vi "Ping.vi"(2 "error in":errorcluster caption="错误输入（无错误）", 3 "NetAdress":string) -> (0 "error out":errorcluster caption="错误输出", 1 "Acess":bool)   [LabVIEW 2013]
panel:
  out "standard output":string caption="标准输出"
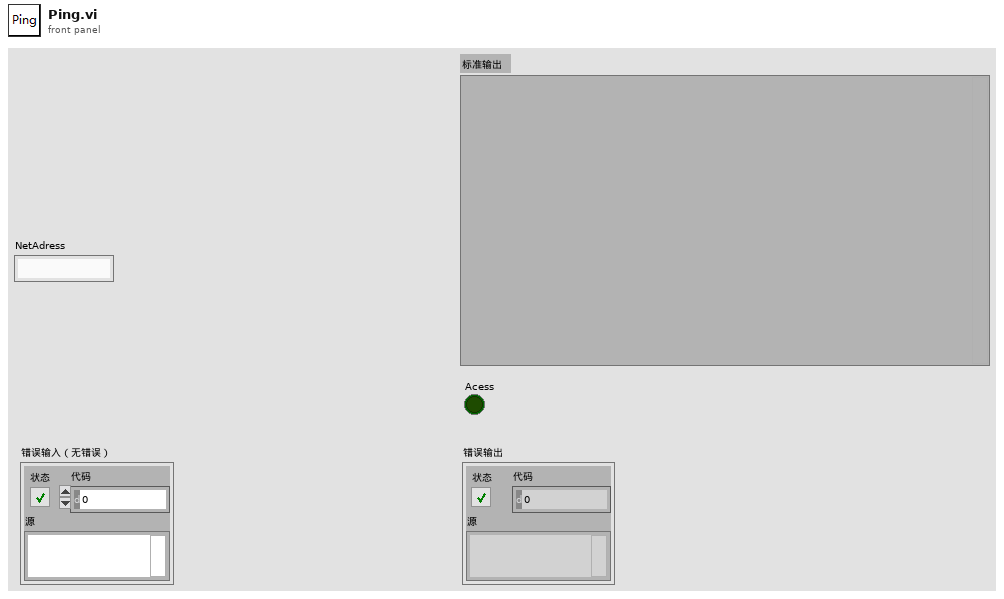
[diagram p1: front panel]
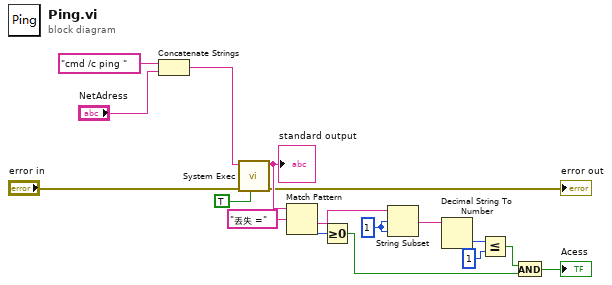
[diagram p0: block diagram]
diagram:
  w12 = 1
  n1 = Concatenate Strings("cmd /c ping " ("command line"), "NetAdress") -> (w1:string)
  n2 = call <vilib>:"System Exec.vi"("run minimized? (F)"=TRUE, "error in (no error)"="error in", "command line"=w1) -> ("error out"=→"error out":errorcluster, "standard output"=w16:string)  [unwired: 5 in, 2 out]
  "standard output" <- w16
  n3 = Match Pattern(string=w16, regular expression="丢失 =" ("正则表达式")) -> (after substring=w13:string, offset past match=w14:i32)  [unwired: 1 in, 2 out]
  n4 = Greater Or Equal To 0?(x=w14) -> (x >= 0?=w7:bool)
  n5 = String Subset(string=w13, offset (0)=w12, length (rest)=w12) -> (substring=w11:string)
  n6 = Decimal String To Number(string=w11) -> (number=w10:i32)  [unwired: 2 in, 1 out]
  n7 = Less Or Equal?(x=w10, y=1) -> (x <= y?=w8:bool)
  n8 = And(x=w8, y=w7) -> (x .and. y?=→"Acess":bool)
